vi "Global_CH375.vi"() -> ()   [LabVIEW 2020]
panel:
  in  "移动速度":u16(ring)=1 items=["1", "1/2", "1/4", "1/8", "1/16", "1/32", "1/64", "1/128"]
  out "当前设备连接状态":bool
  in  "当前角度":dbl
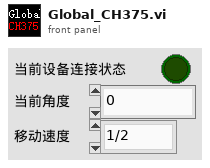
[diagram p1: front panel]
diagram:
